vi "Image_Detect_Object_HQ.vi"(0 "Data":T3={"Pinch-valve"="Test Sample", "XLP 6000 Pump"="MRJ", "Camera1"="", "Camera2"="", "Img_Capt"=FALSE, "Actuator"=FALSE, "Pump"=FALSE, "Cam 1"=FALSE, "Cam 2"=FALSE, "Empty_Refill"=FALSE, "Crop"=FALSE, "Light intensity"=0, "Exposure Time"=0.0, "Sample Name"="", "Operator"="", "Calibration 1"=path "C:/Users/au540322/Desktop/IHS_Project/images/Debris/Debris_0/Debris_0_2019_06_01-23-32-49-686.PNG", "Calibration 2"=path "C:/Users/au540322/Desktop/IHS_Project/images/Debris/Debris_0/Debris_0_2019_06_01-23-32-49-686.PNG", "Framerate"=1, "Timeout Sample"=1, "Collection date"="", "Sample size threshold"=500, "Empty start"=500, "Command"="", "Station"="", "Species Name"="", "Other Notes"="", "Aperture"=enum."Item 3", "Image Process Queue Size"=100, "Image Save Queue Size"=0, "Overload threshold"=0, "Max Framerate"=0, "Rectangle 1"={"Left"=0, "Top"=0, "Right"=0, "Bottom"=0, "Rotation"=0.0}, "Rectangle 2"={"Left"=0, "Top"=100, "Right"=100, "Bottom"=0, "Rotation"=0.0}, "Detection Region %"=200.0, "Detect 1"=path "C:/Users/au540322/Desktop/IHS_Project/images/Debris/Debris_0/Debris_0_2019_06_01-23-32-49-686.PNG", "Detect 2"=path "C:/Users/au540322/Desktop/IHS_Project/images/Debris/Debris_0/Debris_0_2019_06_01-23-32-49-686.PNG", "Max large object threshold"=500, "Open(T)/Close(F)"=FALSE, "Img_Capt Begin"=FALSE, "Dispense Speed"=0, "Flush Size"=0, "Location"="", "Latitude"="", "Longitude"="", "Determiner"="", "Sex"="", "Camera1_Img"=refnum, "Camera2_Img"=refnum, "Img1_Orig_Disp"=refnum, "Img2_Orig_Disp"=refnum, "Img1_Orig_RGB"=refnum, "Img2_Orig_RGB"=refnum, "Blue_Plane_Extract"=refnum, "Subtracted_Plane"=refnum, "Img1_Binary"=refnum, "Img2_Binary"=refnum, "Crop_Mask"=refnum, "Img1_Save"=refnum, "Img2_Save"=refnum, "Img1_Cali_Full"=refnum, "Img2_Cali_Full"=refnum, "Img1_Cali_Detect"=refnum, "Img2_Cali_Detect"=refnum, "Cam 1 queue"=refnum, "Cam 2 queue"=refnum, "Cam 1 - save queue"=refnum, "Cam 2 - save queue"=refnum, "Overlay_Ring"=0, "SystemVersion"=0, "System Serial"="", "Legacy Cam Attributes"=FALSE, "Camera Orientation 1"="", "Camera Orientation 2"="", "Pixel to mm 1"=0.0, "Pixel to mm 2"=0.0, "CAM1 Model"=enum."a2A5328-15ucBAS", "CAM2 Model"=enum."a2A5328-15ucBAS", "Flush Insect"=FALSE, "Pump Size"=FALSE, "Barcode"="", "Phase3"=FALSE, "Mega F3"="", "Container nr."=0.0, "Flush Error"=TRUE, "Start System"=FALSE, "Size Interval"=0.0, "Mun. of containers"=0.0, "Sorting sys."=FALSE, "Initial size"=0.0} {"SystemVersion" items=["Standard", "XL"]; "Overlay_Ring" items=["Session Data", "Extended Setup", "Buffer", "Camera", "Dispenser", "Stats", "Connections"]; "Flush Size" min=1; "Dispense Speed" min=1; "Rectangle 2"."Rotation" format="%.2f"; "Rectangle 2"."Left" scale=0.0..1024.0; "Rectangle 2"."Right" scale=0.0..1024.0; "Rectangle 1"."Rotation" format="%.2f"; "Rectangle 1"."Left" scale=0.0..1024.0; "Rectangle 1"."Right" scale=0.0..1024.0; "Max Framerate" min=1; "Overload threshold" min=1; "Image Save Queue Size" min=1; "Image Process Queue Size" min=1; "Empty start" min=1; "Sample size threshold" min=1; "Framerate" min=1; "Light intensity" scale=0.0..100.0}, 5 "Image Pixels (U32)":u32[][](array[numeric]), 9 "Detect Crop":bool, 12 "Camera":T6=enum."Camera 2") -> (2 "error out":errorcluster, 3 "Obj Size":bool, 4 "Detected object":T1, 6 "Image Out":T1, 8 "Binary":T1, 10 "Object Accept":bool, 14 "ROI descriptor":T2, 15 "Sample Data":dbl[](array[numeric]))   [LabVIEW 2024]
uses:
  Camera_ID.ctl
  controls/Data.ctl
  <vilib>/userDefined/High Color/IMAQdx.ctl
  <vilib>/vision/Image Controls.llb/IMAQ Image.ctl
  <vilib>/vision/NI_Vision_Development_Module.lvlib
panel:
  in  "error in":errorcluster
  in  "Threshold":cluster{"Lower value":sgl, "Upper value":sgl}={"Lower value"=15.0, "Upper value"=256.0} {"Upper value" format="%.2f"; "Lower value" format="%.2f"}
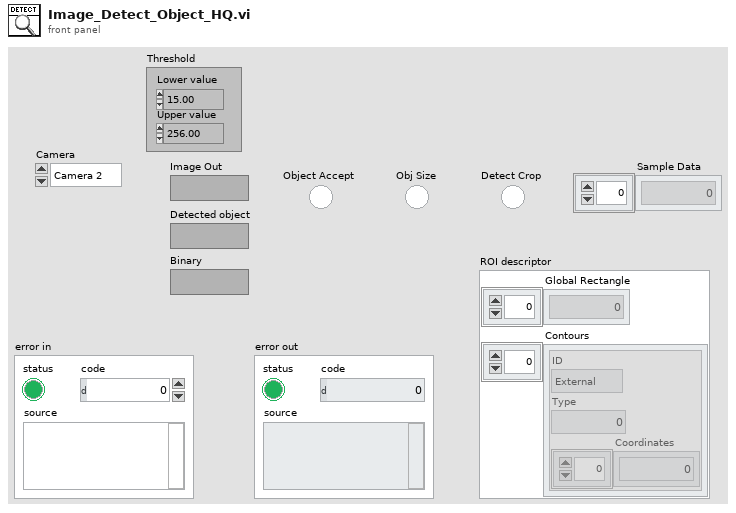
[diagram p1: front panel]
types:
  T1 = typedef "IMAQ Image.ctl" = refnum<image>
  T2 = cluster{"Global Rectangle":i32[], "Contours":cluster{"ID":enum32{"External", "Internal"}, "Type":u32, "Coordinates":i32[]}[]}
  T3 = typedef "Data.ctl" = cluster{"Pinch-valve":refnum<visa-resource-name>, "XLP 6000 Pump":refnum<visa-resource-name>, "Camera1":T4, "Camera2":T4, "Img_Capt":bool, "Actuator":bool, "Pump":bool, "Cam 1":bool, "Cam 2":bool, "Empty_Refill":bool, "Crop":bool, "Light intensity":i32, "Exposure Time":dbl, "Sample Name":string, "Operator":string, "Calibration 1":path, "Calibration 2":path, "Framerate":i32, "Timeout Sample":i32, "Collection date":string, "Sample size threshold":i32, "Empty start":u32, "Command":string, "Station":string, "Species Name":string, "Other Notes":string, "Aperture":enum32{"Item 0", "Item 1", "Item 2", "Item 3"}, "Image Process Queue Size":i32, "Image Save Queue Size":i32, "Overload threshold":i32, "Max Framerate":i32, "Rectangle 1":T5, "Rectangle 2":T5, "Detection Region %":dbl, "Detect 1":path, "Detect 2":path, "Max large object threshold":i32, "Open(T)/Close(F)":bool, "Img_Capt Begin":bool, "Dispense Speed":i32, "Flush Size":i32, "Location":string, "Latitude":string, "Longitude":string, "Determiner":string, "Sex":string, "Camera1_Img":T1, "Camera2_Img":T1, "Img1_Orig_Disp":T1, "Img2_Orig_Disp":T1, "Img1_Orig_RGB":T1, "Img2_Orig_RGB":T1, "Blue_Plane_Extract":T1, "Subtracted_Plane":T1, "Img1_Binary":T1, "Img2_Binary":T1, "Crop_Mask":T1, "Img1_Save":T1, "Img2_Save":T1, "Img1_Cali_Full":T1, "Img2_Cali_Full":T1, "Img1_Cali_Detect":T1, "Img2_Cali_Detect":T1, "Cam 1 queue":refnum<queue>, "Cam 2 queue":refnum<queue>, "Cam 1 - save queue":refnum<queue>, "Cam 2 - save queue":refnum<queue>, "Overlay_Ring":u16, "SystemVersion":u16, "System Serial":string, "Legacy Cam Attributes":bool, "Camera Orientation 1":string, "Camera Orientation 2":string, "Pixel to mm 1":dbl, "Pixel to mm 2":dbl, "CAM1 Model":enum16{"a2A5328-15ucBAS", "acA1920-155uc"}, "CAM2 Model":enum16{"a2A5328-15ucBAS", "acA1920-155uc"}, "Flush Insect":bool, "Pump Size":bool, "Barcode":string, "Phase3":bool, "Mega F3":refnum<visa-resource-name>, "Container nr.":dbl, "Flush Error":bool, "Start System":bool, "Size Interval":dbl, "Mun. of containers":dbl, "Sorting sys.":bool, "Initial size":dbl}
  T4 = typedef "IMAQdx.ctl" = refnum<k21>
  T5 = typedef "IMAQ Rectangle" = cluster{"Left":i32, "Top":i32, "Right":i32, "Bottom":i32, "Rotation":dbl}
  T6 = typedef "Camera_ID.ctl" = enum16{"Camera 1", "Camera 2"}
  T7 = typedef "Particle Parameters" = i32
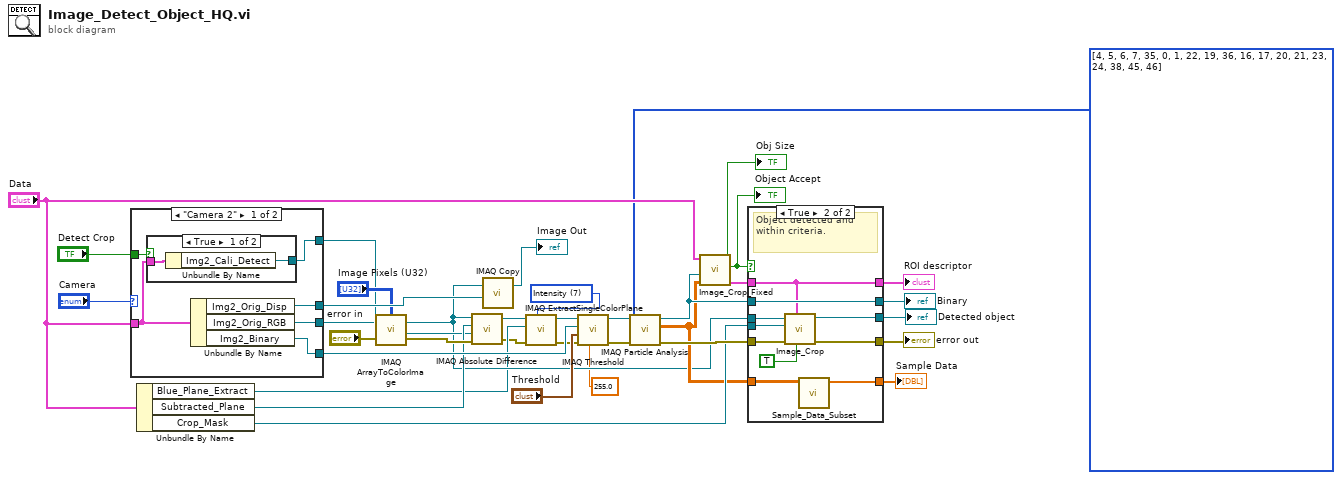
[diagram p0: block diagram]
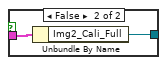
[diagram p2: hidden frame]
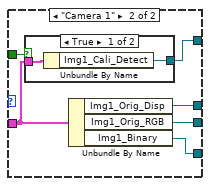
[diagram p3: hidden frame]
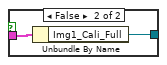
[diagram p4: hidden frame]
diagram:
  w1 = T7[] [4, 5, 6, 7, 35, 0, 1, 22, 19, 36, 16, 17, 20, 21, 23, 24, 38, 45, 46] items=["Center of Mass X", "Center of Mass Y", "First Pixel X", "First Pixel Y", "Bounding Rect Left", "Bounding Rect Top", "Bounding Rect Right", "Bounding Rect Bottom", "Max Feret Diameter Start X", "Max Feret Diameter Start Y", "Max Feret Diameter End X", "Max Feret Diameter End Y", "Max Horiz. Segment Length Left", "Max Horiz. Segment Length Right", "Max Horiz. Segment Length Row", "-", "Bounding Rect Width", "Bounding Rect Height", "Bounding Rect Diagonal", "Perimeter", "Convex Hull Perimeter", "Holes' Perimeter", "Max Feret Diameter", "Equivalent Ellipse Major Axis", "Equivalent Ellipse Minor Axis", "Equivalent Ellipse Minor Axis (Feret)", "Equivalent Rect Long Side", "Equivalent Rect Short Side", "Equivalent Rect Diagonal", "Equivalent Rect Short Side (Feret)", "Average Horiz. Segment Length", "Average Vert. Segment Length", "Hydraulic Radius", "Waddel Disk Diameter", "-", "Area", "Holes' Area", "Particle & Holes' Area", "Convex Hull Area", "Image Area", "-", "Number of Holes", "Number of Horiz. Segments", "Number of Vert. Segments", "-", "Orientation", "Max Feret Diameter Orientation", "-", "% Area/Image Area", "% Area/(Particle & Holes' Area)", "Ratio of Equivalent Ellipse Axes", "Ratio of Equivalent Rect Sides", "-", "Elongation Factor", "Compactness Factor", "Heywood Circularity Factor", "Type Factor", "-", "Sum X", "Sum Y", "Sum XX", "Sum XY", "Sum YY", "Sum XXX", "Sum XXY", "Sum XYY", "Sum YYY", "-", "Moment of Inertia XX", "Moment of Inertia XY", "Moment of Inertia YY", "Moment of Inertia XXX", "Moment of Inertia XXY", "Moment of Inertia XYY", "Moment of Inertia YYY", "Norm. Moment of Inertia XX", "Norm. Moment of Inertia XY", "Norm. Moment of Inertia YY", "Norm. Moment of Inertia XXX", "Norm. Moment of Inertia XXY", "Norm. Moment of Inertia XYY", "Norm. Moment of Inertia YYY", "Hu Moment 1", "Hu Moment 2", "Hu Moment 3", "Hu Moment 4", "Hu Moment 5", "Hu Moment 6", "Hu Moment 7"] ("Pixel Measurements")
  w12 = 7 items=["Red", "Green", "Blue", "Hue", "Saturation", "Luminance", "Value", "Intensity"] ("Color Plane")
  n1 = case shown="\"Camera 2\"" "Camera" {
    tunnel: "Data" -> [w41 w51]
    tunnel: [w40 w50] -> w14
    tunnel: [w38 w49] -> w11
    tunnel: [w39 w47] -> w27
    tunnel: "Detect Crop" -> [w42 w52]
    tunnel: [w37 w48] -> w20
    frame "Camera 2" {
      n2 = case shown="True" w42 {
        tunnel: w41 -> [w44 w46]
        tunnel: [w43 w45] -> w40
        frame True {
          n3 = Unbundle By Name(w44) -> ("Img2_Cali_Detect"=w43:T1)
        }
        frame False {
          n4 = Unbundle By Name(w46) -> ("Img2_Cali_Full"=w45:T1)
        }
      }
      n5 = Unbundle By Name(w41) -> ("Img2_Orig_Disp"=w37:T1, "Img2_Orig_RGB"=w38:T1, "Img2_Binary"=w39:T1)
    }
    frame "Camera 1" {
      n6 = case shown="True" w52 {
        tunnel: w51 -> [w54 w56]
        tunnel: [w53 w55] -> w50
        frame True {
          n7 = Unbundle By Name(w54) -> ("Img1_Cali_Detect"=w53:T1)
        }
        frame False {
          n8 = Unbundle By Name(w56) -> ("Img1_Cali_Full"=w55:T1)
        }
      }
      n9 = Unbundle By Name(w51) -> ("Img1_Orig_Disp"=w48:T1, "Img1_Orig_RGB"=w49:T1, "Img1_Binary"=w47:T1)
    }
  }
  n10 = Unbundle By Name("Data") -> ("Blue_Plane_Extract"=w9:T1, "Subtracted_Plane"=w15:T1, "Crop_Mask"=w28:T1)
  n11 = call "IMAQ ArrayToColorImage"("Image Pixels (U32)"="Image Pixels (U32)", "Image"=w11, "error in (no error)"="error in") -> ("Image Out"=w10:T1, "error out"=w17:errorcluster)  [unwired: 2 in]
  n12 = call "IMAQ Absolute Difference"("Image Src A"=w10, "Image Dst"=w15, "Image Src B"=w14, "error in (no error)"=w17) -> ("Image Dst Out"=w13:T1, "error out"=w7:errorcluster)  [unwired: 3 in]
  n13 = call "IMAQ Copy"("Image Dst"=w20, "Image Src"=w10) -> ("Image Dst Out"=→"Image Out":T1)  [unwired: 4 in, 1 out]
  n14 = call "IMAQ ExtractSingleColorPlane"("Color Plane"=w12, "error in (no error)"=w7, "Image Dst"=w9, "Image Src"=w13) -> ("error out"=w6:errorcluster, "Image Dst Out"=w8:T1)  [unwired: 6 out]
  n15 = call "IMAQ Threshold"("Replace Value"=255.0, "error in (no error)"=w6, "Range"="Threshold", "Image Dst"=w27, "Image Src"=w8) -> ("error out"=w31:errorcluster, "Image Dst Out"=w33:T1)  [unwired: 1 in, 4 out]
  n16 = call "IMAQ Particle Analysis"("error in (no error)"=w31, "Pixel Measurements"=w1, "Image"=w33) -> ("error out"=w34:errorcluster, "Particle Measurements (Pixels)"=w23:dbl[][], "Image Out (duplicate)"=w35:T1)  [unwired: 2 in, 4 out]
  n17 = call "Image_Crop_Fixed.vi"("Particle Measurements"=w23, "Image  in"=w35, "Data"="Data") -> ("ROI descriptor"=w36:T2, "Object accept"=w26:bool, "Object"=→"Obj Size":bool)  [unwired: 6 in]
  "Object Accept" <- w26
  n18 = case shown="True" w26 {
    tunnel: [w57 w68] -> w3
    tunnel: w34 -> [w58 w66]
    tunnel: [w59 w67] -> w4
    tunnel: w35 -> [w59 w67]
    tunnel: [w58 w65] -> w16
    tunnel: w36 -> [_ w61]
    tunnel: w28 -> [_ w60]
    tunnel: w10 -> [w57 w64]
    tunnel: w23 -> [_ w63]
    tunnel: [_ w62] -> w22
    tunnel: [_ w61] -> w18
    frame False {
      # "No object found or not within criteria."
    }
    frame True {
      # "Object detected and within criteria."
      n19 = call "Image_Crop.vi"("Shrink"=TRUE, "ROI Descriptor"=w61, "error in (no error)"=w66, "Image Dest"=w60, "Image Src"=w64) -> ("error out"=w65:errorcluster, "Image Out"=w68:T1)  [unwired: 5 in]
      n20 = call "Sample_Data_Subset.vi"("Particle Measurements (Pixels)"=w63) -> ("Sample Data"=w62:dbl[])  [unwired: 10 in]
    }
  }
  "error out" <- w16
  "Sample Data" <- w22
  "ROI descriptor" <- w18
  "Detected object" <- w3
  "Binary" <- w4
